vi "PriorZstage.vi"() -> ()   [LabVIEW 2021]
uses:
  Prior_Zmotor_class/Prior_Zmotor.lvclass
panel:
  out "Serial Settings:Number of Bytes at Serial Port":u32
  in  "Zero":bool
  in  "Enable Joystick":bool
  in  "VISA resource name":refnum<visa-resource-name>
  in  "Pos (um)":i32
  in  "Go to Pos":bool
  out "IsMoving?":bool
  out "Waveform Chart":dbl(graph)
  in  "stop":bool
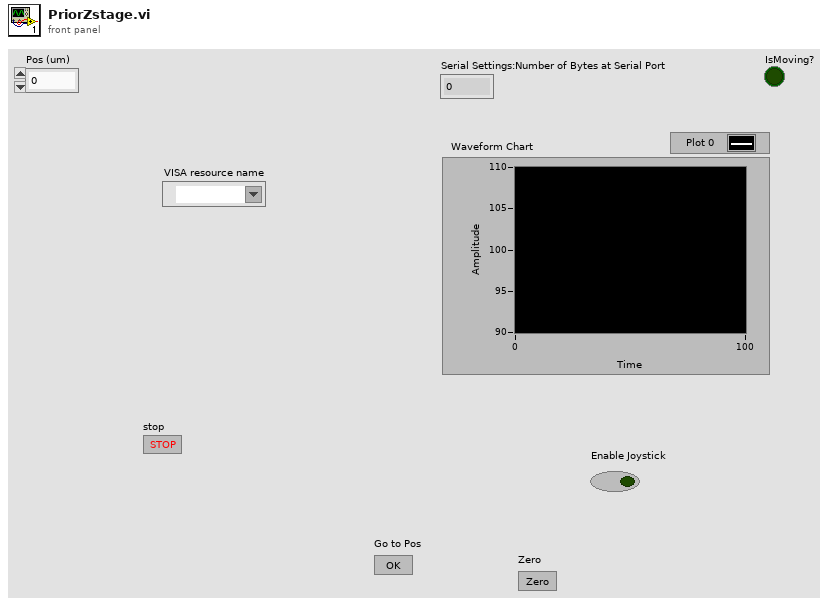
[diagram p1: front panel]
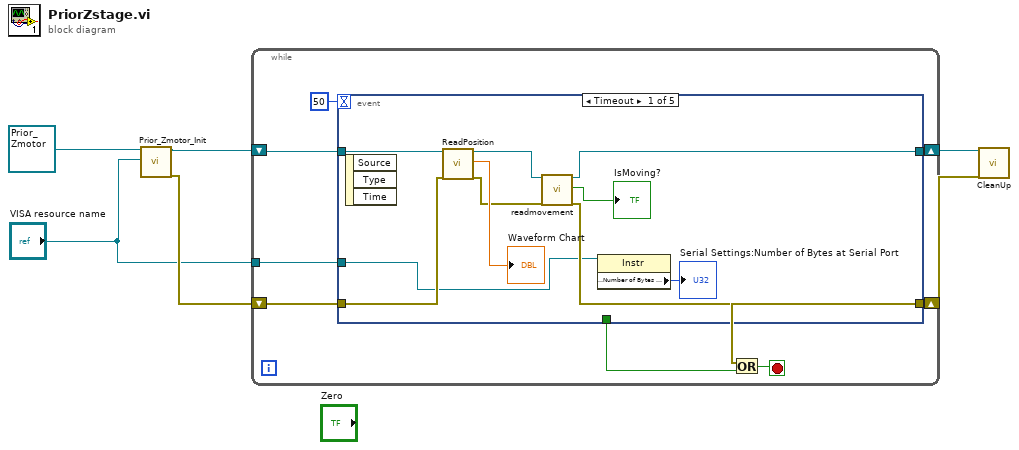
[diagram p0: block diagram]
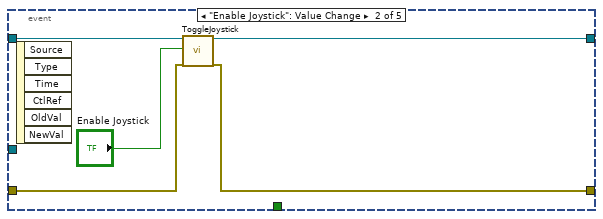
[diagram p2: hidden frame]
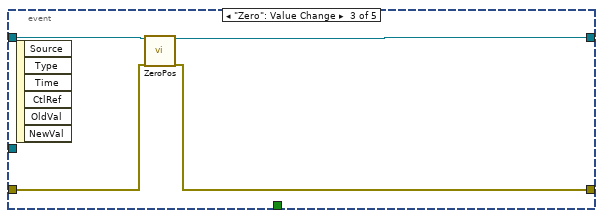
[diagram p3: hidden frame]
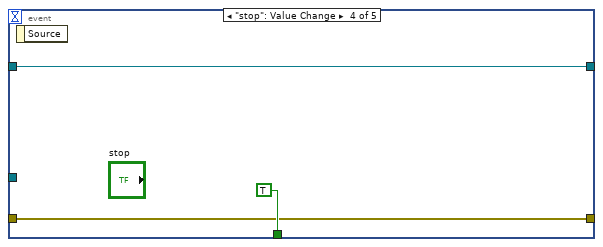
[diagram p4: hidden frame]
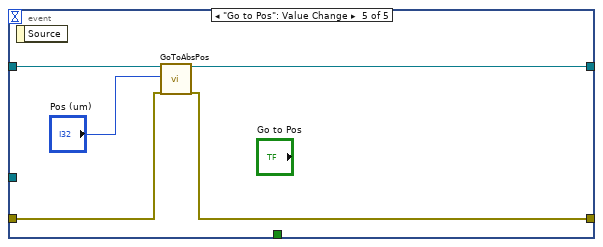
[diagram p5: hidden frame]
diagram:
  n1 = call "Prior_Zmotor_Init.vi"("object in"=refnum<class "Prior_Zmotor.lvclass"> refnum, "VISA resource name"="VISA resource name") -> ("object out"=w3:refnum<class "Prior_Zmotor.lvclass">, "error out"=w5:errorcluster)  [unwired: 16 in]
  n2 = while {
    shift-right: [w11] -> w4
    shift-left: w5 -> [w12]
    shift-right: [w9] -> w2
    shift-left: w3 -> [w10]
    tunnel: "VISA resource name" -> [w7]
    stop <- w14 stop-if-true
    n3 = event shown="[0] Timeout" {
      selector: _ -> [_ _ _ _ _]
      dyn-events: _ -> [_ _ _ _ _]
      timeout: 50 -> [_ _ _ _ _]
      tunnel: [_ _ _ TRUE _] -> w13
      tunnel: w12 -> [w18 w26 w31 w35 w39]
      tunnel: [w17 w25 w30 w35 w38] -> w11
      tunnel: w10 -> [w24 w29 w33 w34 w41]
      tunnel: [w20 w28 w32 w34 w40] -> w9
      tunnel: w7 -> [w16 _ _ _ _]
      event Timeout {
        n4 = event-data() -> ()  [unwired: 1 in, 3 out]
        n5 = call-dynamic "ReadPosition.vi"("object in"=w24, "error in (no error)"=w18) -> ("object out"=w21:refnum<class "Prior_Zmotor.lvclass">, "Position (um)"=→"Waveform Chart":dbl, "error out"=w19:errorcluster)  [unwired: 15 in]
        n6 = call-dynamic "readmovement.vi"("object in"=w21, "error in (no error)"=w19) -> ("object out"=w20:refnum<class "Prior_Zmotor.lvclass">, "IsMoving?"=→"IsMoving?":bool, "error out"=w17:errorcluster)  [unwired: 15 in]
        n7 = property class="Instr"(reference=w16) -> ("Serial Settings:Number of Bytes at Serial Port"=→"Serial Settings:Number of Bytes at Serial Port":u32)  [unwired: 1 in, 2 out]
      }
      event "Enable Joystick": Value Change {
        n8 = event-data() -> ()  [unwired: 1 in, 6 out]
        n9 = call-dynamic "ToggleJoystick.vi"("object in"=w29, "Enable(T)/Disable(F)"="Enable Joystick", "error in (no error)"=w26) -> ("object out"=w28:refnum<class "Prior_Zmotor.lvclass">, "error out"=w25:errorcluster)  [unwired: 15 in]
      }
      event "Zero": Value Change {
        n10 = event-data() -> ()  [unwired: 1 in, 6 out]
        n11 = call-dynamic "ZeroPos.vi"("object in"=w33, "error in (no error)"=w31) -> ("object out"=w32:refnum<class "Prior_Zmotor.lvclass">, "error out"=w30:errorcluster)  [unwired: 16 in]
      }
      event "stop": Value Change {
        n12 = event-data() -> ()  [unwired: 1 in, 1 out]
      }
      event "Go to Pos": Value Change {
        n13 = event-data() -> ()  [unwired: 1 in, 1 out]
        n14 = call-dynamic "GoToAbsPos.vi"("object in"=w41, "Pos (um)"="Pos (um)", "error in (no error)"=w39) -> ("object out"=w40:refnum<class "Prior_Zmotor.lvclass">, "error out"=w38:errorcluster)  [unwired: 14 in, 1 out]
      }
    }
    n15 = Or(x=w11, y=w13) -> (x .or. y?=w14:bool)
  }
  n16 = call-dynamic "CleanUp.vi"("object in"=w2, "error in (no error)"=w4) -> ()  [unwired: 16 in, 2 out]
